vi "test Data Width and Data Loss Error.vi"(8 "error in (no error)":errorcluster, 11 "TestCase in":refnum<class "BNR.lvclass">) -> (0 "error out":errorcluster, 3 "TestCase out":refnum<class "BNR.lvclass">)   [LabVIEW 2027, in "BNR.lvclass"]
uses:
  BNR.lvclass
  aa9375b4-1f31-4778-92c7-5f2d7a262410.vi
  d96fb5d2-e0e4-48b8-8350-325a5946da95.vi
  afef55db-8add-425d-99f2-96b77fef3dec.vi
  66fbdf8c-a380-4cfa-b495-70a8485551d5.vi
  aa9375b4-1f31-4778-92c7-5f2d7a262410.vi/9377bb8f-44b5-4a8f-87f1-966fd5a9edcc.vi
  aa9375b4-1f31-4778-92c7-5f2d7a262410.vi/e95d9d1f-307c-44d6-9f26-c3f519a4990d.vi
  aa9375b4-1f31-4778-92c7-5f2d7a262410.vi/0c23f515-4369-4514-bc3d-4444e6b437b2.vi
  d96fb5d2-e0e4-48b8-8350-325a5946da95.vi/16a2565b-3c16-407b-a626-9da2a3da432e.vi
  afef55db-8add-425d-99f2-96b77fef3dec.vi/9377bb8f-44b5-4a8f-87f1-966fd5a9edcc.vi
  afef55db-8add-425d-99f2-96b77fef3dec.vi/e95d9d1f-307c-44d6-9f26-c3f519a4990d.vi
  afef55db-8add-425d-99f2-96b77fef3dec.vi/0c23f515-4369-4514-bc3d-4444e6b437b2.vi
  66fbdf8c-a380-4cfa-b495-70a8485551d5.vi/9377bb8f-44b5-4a8f-87f1-966fd5a9edcc.vi
  66fbdf8c-a380-4cfa-b495-70a8485551d5.vi/e95d9d1f-307c-44d6-9f26-c3f519a4990d.vi
  66fbdf8c-a380-4cfa-b495-70a8485551d5.vi/0c23f515-4369-4514-bc3d-4444e6b437b2.vi
  C:/Program Files/National Instruments/LabVIEW 2027/vi.lib/addons/_JKI Toolkits/VI Tester/TestCase.llb/TestCase.lvclass
  <vilib>/addons/_JKI Toolkits/VI Tester/TestCase.llb/TestCase.lvclass
panel:
  out "BNR encoded value":bool[](array[boolean])
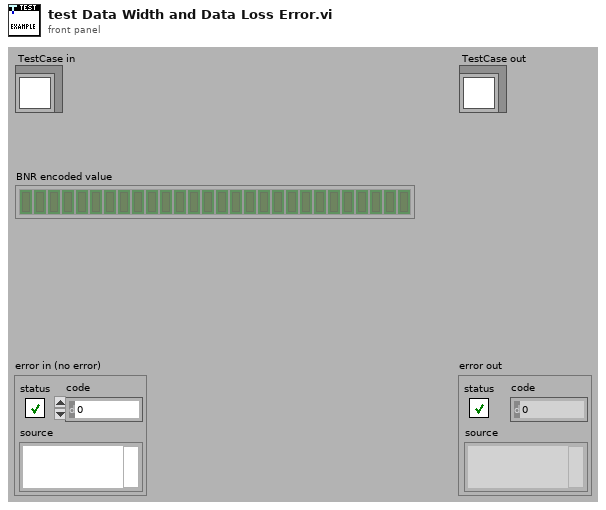
[diagram p1: front panel]
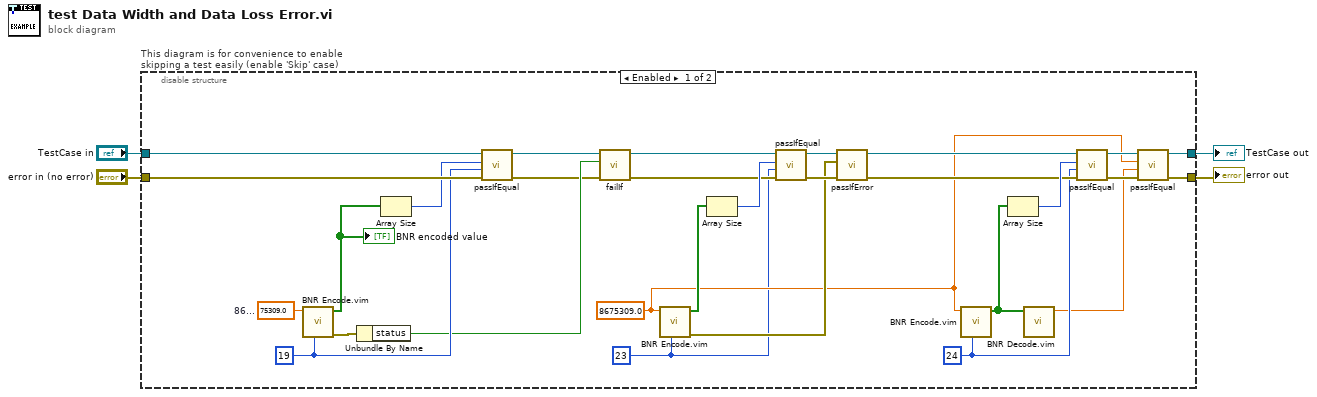
[diagram p0: block diagram]
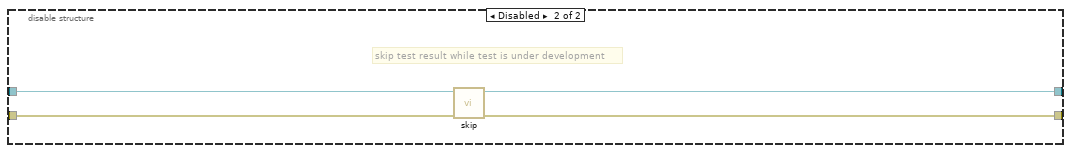
[diagram p2: hidden frame]
diagram:
  n1 = disable-structure "This diagram is for convenience to enable skipping a test easily (enable 'Skip' case)" shown="Enabled" {
    disable-tunnel: "TestCase in" -> [w33 w37]
    disable-tunnel: [w7 w35] -> w4
    disable-tunnel: [w8 w36] -> w1
    disable-tunnel: "error in (no error)" -> [w32 w34]
    frame Enabled {
      w5 = 23 ("data size (bits)")
      w10 = 24 ("data size (bits)")
      w6 = 8675309.0 ("86...")
      w25 = 19 ("data size (bits)")
      w27 = 75309.0  # 86...
      n2 = call "BNR Encode.vim"("data size (bits)"=w25, "value"=w27) -> ("error out"=w22:errorcluster, "BNR encoded value"=w29:bool[])  [unwired: 8 in]
      "BNR encoded value" <- w29
      n3 = Unbundle By Name(w22) -> ("status"=w21:bool)
      n4 = Array Size(array=w29) -> (size(s)=w28:i32)
      n5 = call-dynamic "passIfEqual.vi"("error in (no error)"=w32, "y"=w25, "x"=w28, "TestCase in"=w33) -> ("error out"=w19:errorcluster, "TestCase out"=w20:refnum<class "BNR.lvclass">)  [unwired: 6 in]
      n6 = call-dynamic "failIf.vi"("error in (no error)"=w19, "fail"=w21, "TestCase in"=w20) -> ("error out"=w17:errorcluster, "TestCase out"=w18:refnum<class "BNR.lvclass">)  [unwired: 7 in]
      n7 = call "BNR Encode.vim"("data size (bits)"=w5, "value"=w6) -> ("error out"=w23:errorcluster, "BNR encoded value"=w26:bool[])  [unwired: 8 in]
      n8 = Array Size(array=w26) -> (size(s)=w24:i32)
      n9 = call-dynamic "passIfEqual.vi"("error in (no error)"=w17, "y"=w5, "x"=w24, "TestCase in"=w18) -> ("error out"=w30:errorcluster, "TestCase out"=w31:refnum<class "BNR.lvclass">)  [unwired: 6 in]
      n10 = call-dynamic "passIfError.vi"("error in (no error)"=w30, "error"=w23, "TestCase in"=w31) -> ("error out"=w13:errorcluster, "TestCase out"=w11:refnum<class "BNR.lvclass">)  [unwired: 7 in]
      n11 = call "BNR Encode.vim"("data size (bits)"=w10, "value"=w6) -> ("BNR encoded value"=w12:bool[])  [unwired: 8 in, 1 out]
      n12 = Array Size(array=w12) -> (size(s)=w16:i32)
      n13 = call "BNR Decode.vim"("BNR encoded value"=w12) -> ("value"=w9:dbl)  [unwired: 10 in]
      n14 = call-dynamic "passIfEqual.vi"("error in (no error)"=w13, "y"=w10, "x"=w16, "TestCase in"=w11) -> ("error out"=w15:errorcluster, "TestCase out"=w14:refnum<class "BNR.lvclass">)  [unwired: 6 in]
      n15 = call-dynamic "passIfEqual.vi"("error in (no error)"=w15, "y"=w9, "x"=w6, "TestCase in"=w14) -> ("error out"=w8:errorcluster, "TestCase out"=w7:refnum<class "BNR.lvclass">)  [unwired: 6 in]
    }
    frame Disabled {
      # "skip test result while test is under development"
      n16 = call <vilib>:"skip.vi"("error in (no error)"=w34, "TestCase in"=w37) -> ("error out"=w36:errorcluster, "TestCase out"=w35:refnum<class "BNR.lvclass">)  [unwired: 8 in]
    }
  }
  "error out" <- w1
  "TestCase out" <- w4
